vi "MAN_Query.vi"(0 "System no.":i32=1 min=1 max=4 step=1, 2 "Command":string, 5 "error in":errorcluster) -> (14 "Online Manual":string, 19 "error out":errorcluster)   [LabVIEW 2020]
doc: "Returns online manual entry for given command.\n\nC-867, Mercury_GCS:"
panel:
  # "Returns online manual entry for given command."
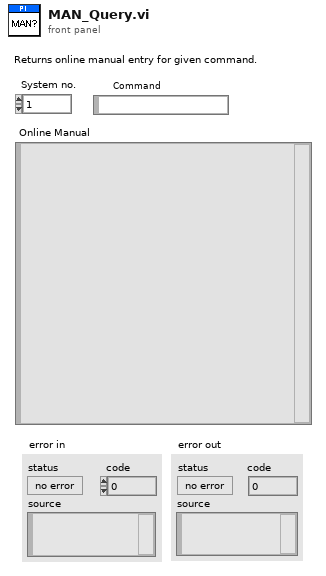
[diagram p1: front panel]
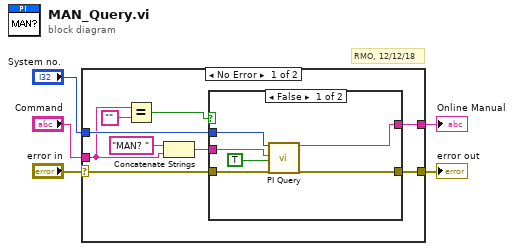
[diagram p0: block diagram]
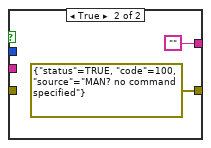
[diagram p2: hidden frame]
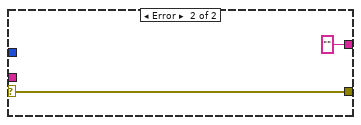
[diagram p3: hidden frame]
diagram:
  # "RMO, 12/12/18"
  n1 = case shown="No Error" "error in" {
    selector: "error in" -> [w6 w23]
    tunnel: [w14 "" ("String read")] -> w5
    tunnel: [w13 w23] -> w4
    tunnel: "System no." -> [w12 _]
    tunnel: "Command" -> [w9 _]
    frame No Error {
      n2 = Equal?(x=w9, y="") -> (x = y?=w11:bool)
      n3 = Concatenate Strings("MAN? " ("string"), w9) -> (w7:string)
      n4 = case shown="False" w11 {
        tunnel: [w16 ""] -> w14
        tunnel: [w15 errorcluster {"status"=TRUE, "code"=100, "source"="MAN? no command specified"} ("error out")] -> w13
        tunnel: w12 -> [w18 _]
        tunnel: w6 -> [w19 _]
        tunnel: w7 -> [w17 _]
        frame False {
          n5 = call "PI Query.vi"("System no."=w18, "String to send"=w17, "Attach termination char.?"=TRUE ("Attach Linefeed?"), "error in"=w19) -> ("String read"=w16:string, "error out"=w15:errorcluster)  [unwired: 3 in, 11 out]
        }
        frame True {
        }
      }
    }
    frame Error {
    }
  }
  "Online Manual" <- w5
  "error out" <- w4
